vi "createTelemetryDynamicData.vi"(8 "error in (no error)":errorcluster, 11 "UserEvents in":refnum<class "UserEvents.lvclass">) -> (0 "error out":errorcluster, 3 "UserEvents out":refnum<class "UserEvents.lvclass">)   [LabVIEW 2016, in "UserEvents.lvclass"]
uses:
  UserEvents.lvclass
  DataTypes/Topics/TelemetryDynamicData.ctl
  DataTypes/Topics/Parts/Timestamp.ctl
  UserEvents.lvclass/UserEvents.ctl
  DataTypes/Topics/M1M3SupportTopics.lvlib
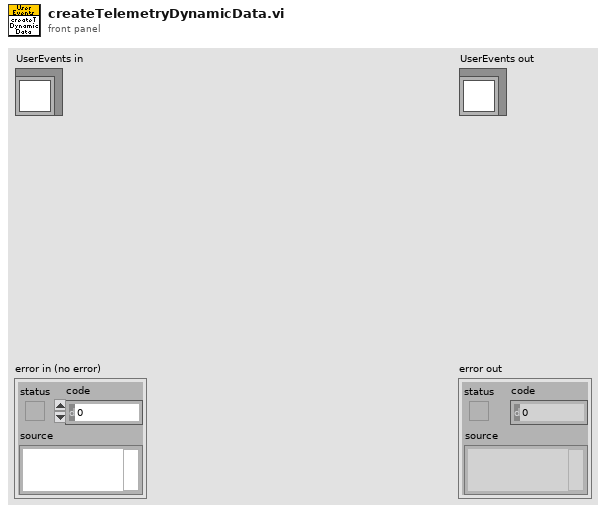
[diagram p1: front panel]
types:
  T1 = typedef "M1M3SupportTopics.lvlib/TelemetryDynamicData.ctl" = cluster{"Timestamp":T2, "AzimuthVelocity":dbl, "ElevationVelocity":dbl, "AzimuthAcceleration":dbl, "ElevationAcceleration":dbl}
  T2 = typedef "M1M3SupportTopics.lvlib/Timestamp.ctl" = dbl
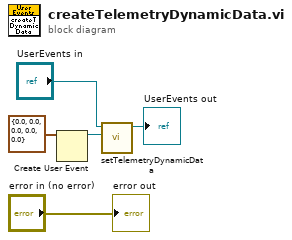
[diagram p0: block diagram]
diagram:
  n1 = Create User Event(user event datatype=T1 {"Timestamp"=0.0, "AzimuthVelocity"=0.0, "ElevationVelocity"=0.0, "AzimuthAcceleration"=0.0, "ElevationAcceleration"=0.0} ("TelemetryDynamicData")) -> (user event=w1:refnum<user-event>)  [unwired: 1 in, 1 out]
  n2 = call "setTelemetryDynamicData.vi"("TelemetryDynamicData"=w1, "UserEvents in"="UserEvents in") -> ("UserEvents out"=→"UserEvents out":refnum<class "UserEvents.lvclass">)  [unwired: 9 in]
  "error out" <- "error in (no error)"
